vi "PID (gain schedule).vi"(0 "gain scheduling variable":dbl format="%.2f", 4 "iteration":i32, 6 "options":T2={"sp low"=0.0, "sp high"=100.0, "out low"=-100.0, "out high"=100.0, "hold (F)"=FALSE, "auto (T)"=TRUE, "pro. band (F)"=FALSE, "reverse acting (T)"=TRUE, "beta"=1.0, "linearity"=1.0, "dt (s)"=-1.0} {"dt (s)" format="%.2f"; "linearity" min=0.0 max=1.0 format="%.2f"; "sp low" format="%.2f"; "sp high" format="%.2f"; "out low" format="%.2f"; "out high" format="%.2f"; "beta" min=0.0 max=1.0 format="%.2f"}, 8 "manual control":dbl format="%.2f", 9 "gain scheduling":T1={"gain schedule"=[100.0], "PID parameters"=[{"Kc"=4.851751673610237, "Ti (min)"=0.021111111111111112, "Td (min)"=0.005277777777777778}], "scheduling input"=0} {"scheduling input" items=["Setpoint", "Process variable", "Controller output", "Gain scheduling input"]; "PID parameters"."Td (min)" format="%.4f"; "PID parameters"."Ti (min)" format="%.4f"; "PID parameters"."Kc" format="%.4f"; "gain schedule" format="%.2f"}, 10 "process variable":dbl format="%.2f", 11 "setpoint":dbl format="%.2f") -> (3 "output":dbl format="%.2f")   [LabVIEW 2020, in "NI_PID__prctrl compat.lvlib"]
doc: "This VI is used to implement a gain schedule for the proportional gain, integral time, and derivative time. Either the setpoint, process variable, controller output, or a user provided value can be used as the scheduling variable.\n\nDescription of the PID algorithm:\n\nDerivative action is on the process variable only. Anti-reset windup and bumpless transfer are supported.\n\nThis VI should be called from inside a while loop with a fixed cycle time. If Cycle Time is less than or equal to zero, an internal timer with 1 millisecond resolution is used for calculations.\n\nThis VI is reentrant, so you can call it from multiple, independent higher-level VIs without interference.\n\nThe default variable ranges correspond to setpoint, process variable, and output expressed in percent. Reverse action (also called increase-decrease) is the \"normal\" controller mode where the output decreases if the process variable is higher than the setpoint.\n\nSwitching from auto to manual is bumpless; the initial value of the Manual Output control is subtracted out so that it is really a \"relative\" output control. Switching from manual to auto is also bumpless.\n\nSwitching to Hold causes the controller to ignore further changes in the process variable and suspends any integral action. Thus, the output stays constant at the last value."
uses:
  NI_PID__prctrl compat.lvlib
panel:
  # "hold (F): default FALSE, no hold.\nauto (T): default TRUE, PID controlling.\npro.band(F): default FALSE, Gain is expressed in actual gain.\n     if TRUE, the proportional band is used.  The relationship \n     between proportional band and gain is gain=100/pro. band\nreverse acting (T): default TRUE, reverse acting. In reverse \n     acting, controller output increases when sp-pv increases.\nsp & pv range: setpoint and process variable range.  Can\n     be either in percentage or actual engineering units.\noutput range: controller output range.  Can be either in\n     percentage or actual engineering units.\nbeta: default 1.0. smaller beta reduces the overshoot in   \n     setpoint response.\nmanual control: when auto is FALSE, controller output =\n     manual control.\nlinearity: default 1.0, linear control action. smaller value \n     reduces controller gain when PV is close to SP."
  # "PID Controller"
  # "SP & PV range:"
  # "Output range:"
  # "-1: default,using\nsystem clock"
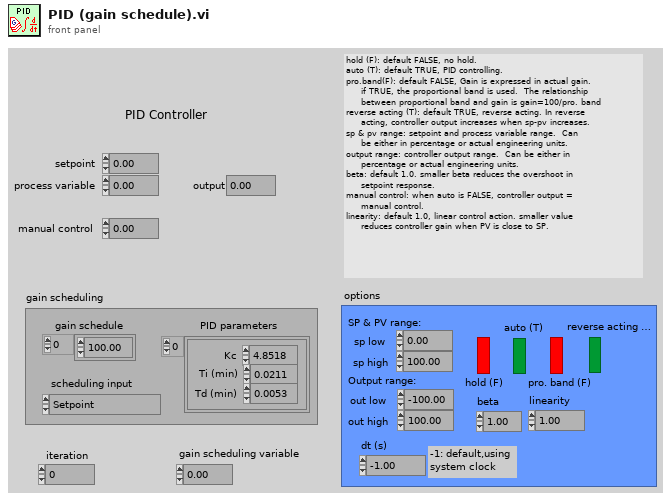
[diagram p1: front panel]
types:
  T1 = cluster{"gain schedule":dbl[], "PID parameters":cluster{"Kc":dbl, "Ti (min)":dbl, "Td (min)":dbl}[], "scheduling input":u16}
  T2 = cluster{"sp low":dbl, "sp high":dbl, "out low":dbl, "out high":dbl, "hold (F)":bool, "auto (T)":bool, "pro. band (F)":bool, "reverse acting (T)":bool, "beta":dbl, "linearity":dbl, "dt (s)":dbl}
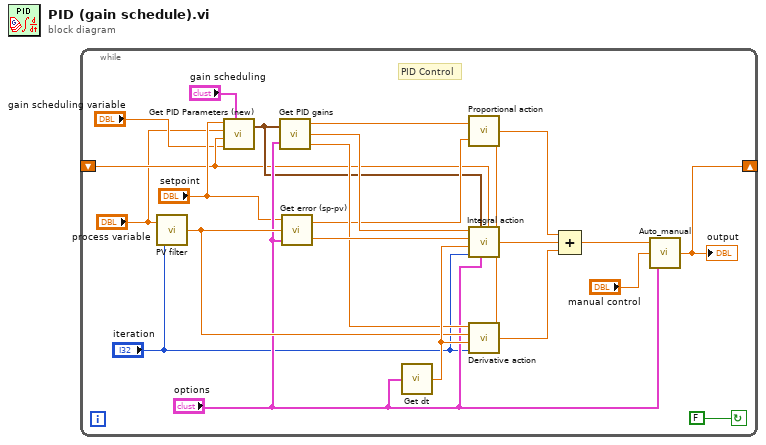
[diagram p0: block diagram]
diagram:
  n1 = while {
    shift-left: _ -> [w5]
    shift-right: [w8] -> _
    stop <- FALSE continue-if-true
    # "PID Control"
    n2 = call "PV filter.vi"("iteration"="iteration", "process variable"="process variable") -> ("filtered pv"=w18:dbl)
    n3 = call "Get PID Parameters (new).vi"("setpoint"="setpoint", "process variable"="process variable", "controller output"=w5, "gain scheduling input"="gain scheduling variable", "gain scheduling"="gain scheduling") -> ("PID parameters"=w7:cluster{"Kp":dbl, "Ti":dbl, "Td":dbl})  [unwired: 1 out]
    n4 = call "Get PID gains.vi"("PID parameters"=w7, "options"="options") -> ("Kc"=w14:dbl, "Ki"=w15:dbl, "Kd"=w16:dbl)
    n5 = call "Get error (sp-pv).vi"("options"="options", "process variable"=w18, "setpoint"="setpoint") -> ("error"=w17:dbl, "error (with beta)"=w13:dbl)
    n6 = call "Get dt.vi"("options"="options") -> ("dt (min.)"=w19:dbl)
    n7 = call "Proportional action.vi"("error"=w13, "Kc"=w14) -> ("proportional action"=w22:dbl)
    n8 = call "Derivative action.vi"("iteration"="iteration", "dt"=w19, "process variable"=w18, "Kd"=w16) -> ("derivative action"=w21:dbl)
    n9 = call "Integral action.vi"("derivative action"=w21, "proportional action"=w22, "prev. control output"=w5, "options"="options", "PID parameters"=w7, "iteration"="iteration", "dt"=w19, "error"=w17, "Ki"=w15) -> ("integral action"=w20:dbl)  [unwired: 2 out]
    n10 = Compound Arithmetic op=ADD(w22, w20, w21) -> (w12:dbl)
    n11 = call "Auto_manual.vi"("options"="options", "manual control"="manual control", "auto control"=w12) -> ("output"=w8:dbl)
    "output" <- w8
  }
